vi "Close_Test.vi"(8 "error in (no error)":errorcluster caption="entrée d'erreur (pas d'erreur)", 11 "Test (Default) en entrée":refnum<class "Sequencer (Default).lvclass">) -> (0 "error out":errorcluster caption="sortie d'erreur", 3 "Test (Default) en sortie":refnum<class "Sequencer (Default).lvclass">)   [LabVIEW 2020, in "Library Core.lvlib" / "Sequencer (Default).lvclass"]
uses:
  Sequencer (Default).lvclass
  Sequencer (Default).lvclass/Sequencer (Default).ctl
  <vilib>/ActorFramework/Message Enqueuer/Message Enqueuer.lvclass/Message Enqueuer.ctl
  Commun VI/TypeDef/Commande Test/Commande Data Test.ctl
  Commun VI/TypeDef/Commande Test/Commande Value Type.ctl
  Commun VI/TypeDef/Commande Test/Commande Type Test.ctl
  Log File/Class Log_File Altyor/Class Log_File Altyor.lvclass
  C:/Users/ngarcin/OneDrive - Altyor/Standard TB/Class/Log File/Log_File (Default)/Class Log_File (Default).lvclass
  JSON API/JSON Value/Set from JSON string.vi
  <vilib>/ActorFramework/Message Enqueuer/Enqueue.vi
  <vilib>/ActorFramework/Stop Msg/Stop Msg.lvclass
  C:/Program Files (x86)/National Instruments/LabVIEW 2020/vi.lib/ActorFramework/Message/Message.lvclass
  <vilib>/ActorFramework/Message Priority Queue/Priority Enqueue.vi
  JSON API/Variant JSON/Variant to JSON.vi
  JSON API/JSON Value/Get Item by name array.vi
  JSON API/JSON Value/JSON Value.lvclass
  Instrument/Instrument (Default)/Class Instrument (Default).lvclass
  Commun VI/Library Commun.lvlib
  JSON API/Get Polymorphic/JSON GetSet.lvlib
  JSON API/Variant JSON/Variant JSON.lvlib
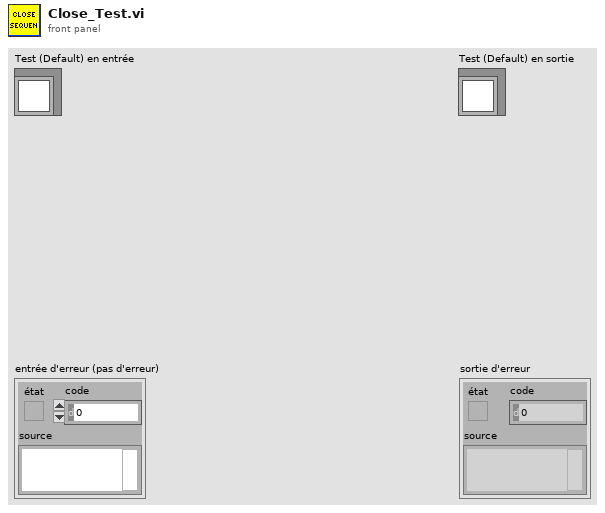
[diagram p1: front panel]
types:
  T1 = enum16{"Add Instr", "Remove Instr", "List Instr", "Get Instr Class", "Get Instr obj", "Save Insrt obj", "Modify Insrt obj", "Init"}
  T2 = enum16{"Init", "Add Actor", "Delete Actor", "Get Actor Queue", "Get Log Actor Queue", "List all actors"}
  T3 = cluster{"Path_Log_File":path, "Delimit":string, "File For Save":refnum<queue>, "Event Error":refnum<user-event>, "Class Log_File":refnum<class "Class Log_File Altyor.lvclass">}
  T4 = cluster{"Name":string, "Instrument":refnum<class "Class Instrument (Default).lvclass">, "Close After Autotest":bool}[]
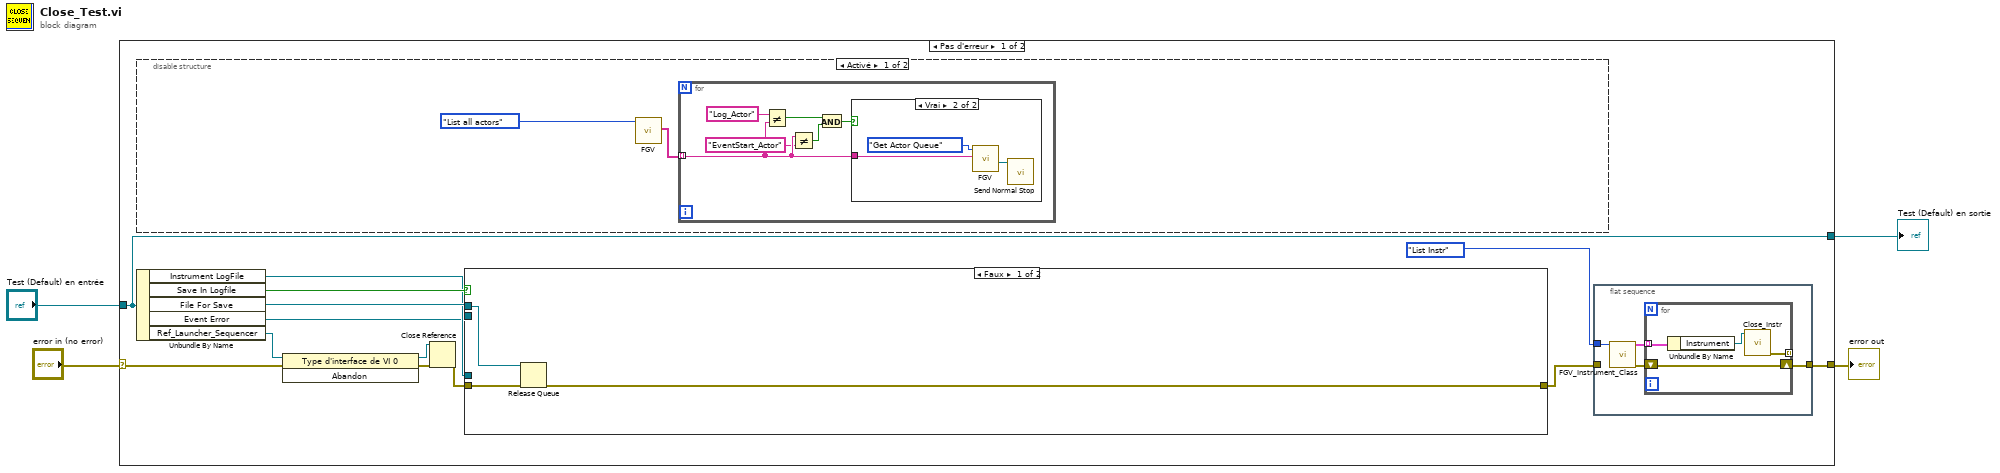
[diagram p0: block diagram]
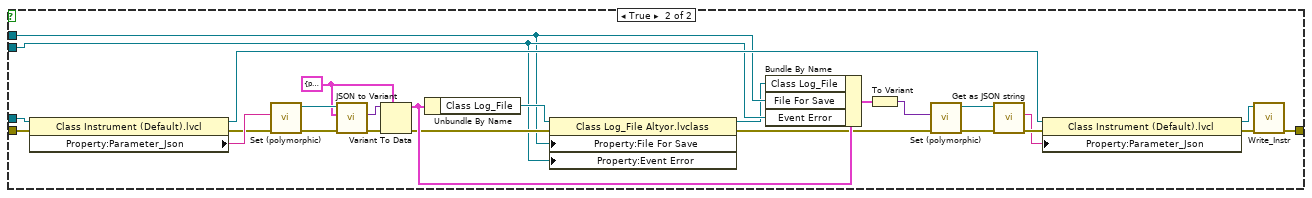
[diagram p4: hidden frame]
diagram:
  n1 = case shown="Pas d'erreur" "error in (no error)" {
    selector: "error in (no error)" -> [w13 w67]
    tunnel: [w7 w67] -> w2
    tunnel: [w15 w66] -> w3
    tunnel: "Test (Default) en entrée" -> [w15 w66]
    frame No Error {
      n2 = disable-structure shown="Activé" {
        frame Enabled {
          n3 = call "FGV.vi"("Action"=T2."List all actors") -> ("Actor names"=w26:string[])  [unwired: 8 in, 2 out]
          n4 = for {
            tunnel: w26 -> [w30] mode=indexing
            n5 = Not Equal?(x="Log_Actor" ("Actor name"), y=w30) -> (x != y?=w33:bool)
            n6 = Not Equal?(x=w30, y="EventStart_Actor" ("Actor name")) -> (x != y?=w29:bool)
            n7 = Compound Arithmetic op=AND ("Opérateur arithmétique")(w33, w29) -> (w31:bool)
            n8 = case shown="Vrai" w31 {
              tunnel: w30 -> [_ w36]
              frame False {
              }
              frame True {
                n9 = call "FGV.vi"("Actor name"=w36, "Action"=T2."Get Actor Queue") -> ("Actor's Queue Out"=w34:refnum<class "Message Enqueuer.lvclass">)  [unwired: 7 in, 2 out]
                n10 = call <vilib>:"Send Normal Stop.vi"("Message Enqueuer"=w34) -> ()  [unwired: 10 in, 1 out]
              }
            }
          }
        }
        frame Disabled {
        }
      }
      n11 = Unbundle By Name(w15) -> ("Instrument LogFile"=w9:refnum<class "Class Instrument (Default).lvclass">, "Save In Logfile"=w10:bool, "File For Save"=w16:refnum<queue>, "Event Error"=w8:refnum<user-event>, "Ref_Launcher_Sequencer"=w14:refnum<vi>)
      n12 = invoke class="Type d'interface de VI 0" method="Abandon"(reference=w14, error in=w13) -> (reference out=w12:refnum<vi>, error out=w11:errorcluster)  [unwired: 1 in, 1 out]
      n13 = Close Reference(reference=w12, error in (no error)=w11) -> (error out=w17:errorcluster)
      n14 = case shown="Faux" w10 {
        tunnel: w17 -> [w39 w63]
        tunnel: w16 -> [w38 w41]
        tunnel: [w37 w65] -> w6
        tunnel: w9 -> [_ w64]
        tunnel: w8 -> [_ w42]
        frame False {
          n15 = Release Queue(queue=w38, error in (no error)=w39) -> (error out=w37:errorcluster)  [unwired: 1 in, 2 out]
        }
        frame True {
          w54 = T3 {"Path_Log_File"=path "", "Delimit"="", "File For Save"=refnum, "Event Error"=refnum, "Class Log_File"=refnum} ("Parameter")
          n16 = property class="Class Instrument (Default).lvcl"(reference=w64, error in=w63) -> (reference out=w62:refnum<class "Class Instrument (Default).lvclass">, error out=w52:errorcluster, "Property:Parameter_Json"=w53:string)
          n17 = call-poly "Set (polymorphic).vi"("error in (no error)"=w52, "JSON stream"=w53) -> ("error out"=w56:errorcluster, "JSON Value out"=w58:refnum<class "JSON Value.lvclass">)  [unwired: 7 in, 1 out]
          n18 = call "JSON to Variant.vi"("error in (no error)"=w56, "Variant (Data Type)"=w54, "JSON Value"=w58) -> ("error out"=w57:errorcluster, "Variant out"=w55:variant)  [unwired: 7 in]
          n19 = Variant To Data(error in=w57, type=w54, Variant=w55) -> (data=w46:T3, error out=w45:errorcluster)
          n20 = Unbundle By Name(w46) -> ("Class Log_File"=w43:refnum<class "Class Log_File Altyor.lvclass">)
          n21 = property class="Class Log_File Altyor.lvclass"(reference=w43, error in=w45, "Property:File For Save"=w41, "Property:Event Error"=w42) -> (reference out=w40:refnum<class "Class Log_File Altyor.lvclass">, error out=w44:errorcluster)
          n22 = Bundle By Name(cluster=w46, "Class Log_File"=w40, "File For Save"=w41, "Event Error"=w42) -> (w51:T3)
          n23 = To Variant(anything=w51) -> (Variant=w61:variant)
          n24 = call-poly "Set (polymorphic).vi"("error in (no error)"=w44, "Variant"=w61) -> ("error out"=w59:errorcluster, "JSON Value out"=w60:refnum<class "JSON Value.lvclass">)  [unwired: 8 in]
          n25 = call "Get as JSON string.vi"("error in (no error)"=w59, "JSON Value in"=w60) -> ("error out"=w50:errorcluster, "<JSON>"=w47:string)  [unwired: 8 in]
          n26 = property class="Class Instrument (Default).lvcl"(reference=w62, error in=w50, "Property:Parameter_Json"=w47) -> (reference out=w48:refnum<class "Class Instrument (Default).lvclass">, error out=w49:errorcluster)
          n27 = call-dynamic "Write_Instr.vi"("error in (no error)"=w49, "Class Multimeter (Default) en entrée"=w48) -> ("error out"=w65:errorcluster)  [unwired: 8 in, 1 out]
        }
      }
      n28 = flat-sequence {
        tunnel: T1."List Instr" ("Action") -> [w21]
        tunnel: [w18] -> w7
        tunnel: w6 -> [_]
        frame #0 {
          n29 = call "FGV_Instrument_Class.vi"("Action"=w21) -> ("Instruments 2"=w20:T4, "error out"=w19:errorcluster)  [unwired: 12 in, 1 out]
          n30 = for {
            tunnel: w20 -> [w25] mode=indexing
            shift-right: [w24] -> w18
            shift-left: w19 -> [w24]
            tunnel: [w22] -> _ mode=indexing
            n31 = Unbundle By Name(w25) -> ("Instrument"=w23:refnum<class "Class Instrument (Default).lvclass">)
            n32 = call-dynamic "Close_Instr.vi"("Class Instrument (Default) en entrée"=w23) -> ("error out"=w22:errorcluster)  [unwired: 9 in, 1 out]
          }
        }
      }
    }
    frame Error {
    }
  }
  "error out" <- w2
  "Test (Default) en sortie" <- w3
